vi "Setting the highest AC voltage.vi"(2 "Assign  averexp according to the chart on the right":dbl=1.0, 3 "VISA resource name":refnum<visa-resource-name>="GPIB12::28::INSTR") -> (0 "Read out result":string="UC= 9456.092   PF L= 658.76     NS V=0.10   V\r\n", 1 "Send string":string="UNITS 1;\nSHOW UN")   [LabVIEW 2010]
panel:
  in  "byte count":u32=128
  out "error out":errorcluster {"code" format="%.0x"}
  in  "error in":errorcluster {"code" format="%.0x"}
  # "Set the highest AC voltage limit"
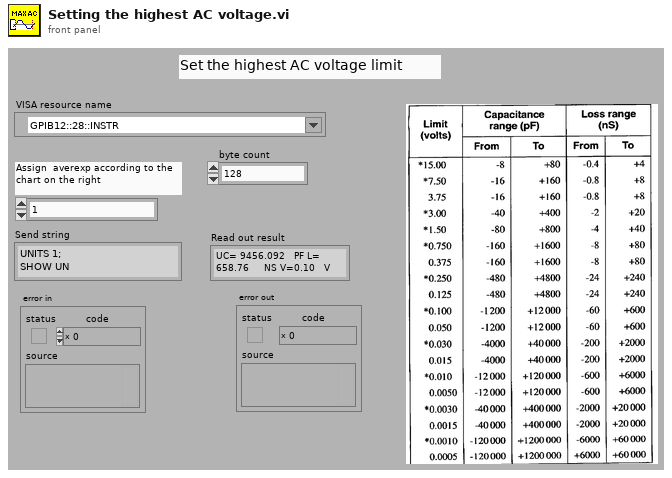
[diagram p1: front panel]
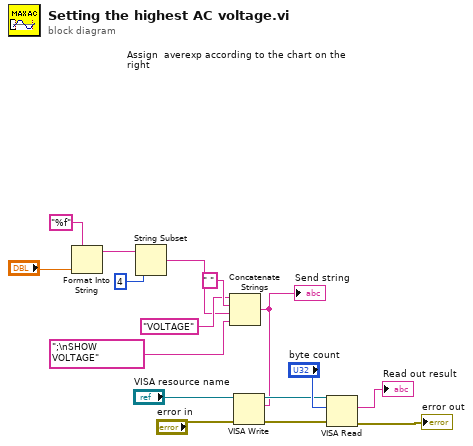
[diagram p0: block diagram]
diagram:
  n1 = Format Into String(format string="%f", "Assign  averexp according to the chart on the right") -> (resulting string=w4:string)  [unwired: 2 in, 1 out]
  n2 = String Subset(string=w4, length (rest)=4 ("length (rest)")) -> (substring=w2:string)  [unwired: 1 in]
  n3 = Concatenate Strings("VOLTAGE" ("string"), " " ("string"), w2, ";\nSHOW VOLTAGE" ("format string")) -> (w7:string)
  "Send string" <- w7
  n4 = VISA Write(VISA resource name="VISA resource name", write buffer=w7, error in (no error)="error in") -> (VISA resource name out=w10:refnum<visa-resource-name>, error out=w9:errorcluster)  [unwired: 1 out]
  n5 = VISA Read(VISA resource name=w10, byte count="byte count", error in (no error)=w9) -> (read buffer=→"Read out result":string, error out=→"error out":errorcluster)  [unwired: 2 out]
